vi "SLM 10-bit to 2xSLM 8-bit.vi"(1 "Array of voltages":i32[](array[numeric])) -> (0 "Array of SLM accepted voltages":u8[](array[numeric]))   [LabVIEW 2022 SP3]
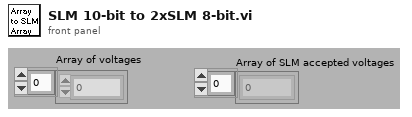
[diagram p1: front panel]
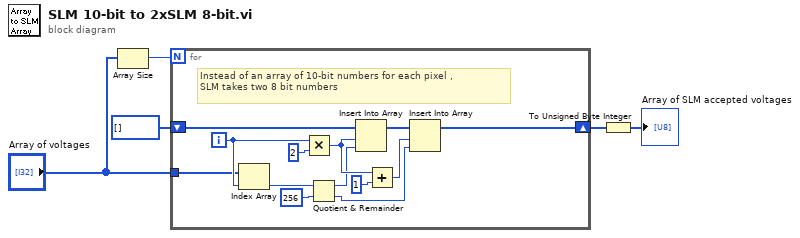
[diagram p0: block diagram]
diagram:
  n1 = Array Size(array="Array of voltages") -> (size(s)=w1:i32)
  n2 = for {
    N: w1 -> [_]
    shift-right: [w15] -> w4
    shift-left: i32[] [] -> [w18]
    tunnel: "Array of voltages" -> [w7]
    i -> [w9]
    # "Instead of an array of 10-bit numbers for each pixel ,\nSLM takes two 8 bit numbers"
    n3 = Index Array(array=w7, index=w9) -> (element=w6:i32)
    n4 = Multiply(x=w9, y=2) -> (x*y=w11:i32)
    n5 = Quotient & Remainder(x=w6, y=u16 256) -> (x-y*floor(x/y)=w8:i32, floor(x/y)=w10:i32)
    n6 = Insert Into Array(array=w18, index=w11, new element=w8) -> (w16:i32[])
    n7 = Add(x=w11, y=1) -> (x+y=w13:i32)
    n8 = Insert Into Array(array=w16, index=w13, new element=w10) -> (w15:i32[])
  }
  n9 = To Unsigned Byte Integer(number=w4) -> (unsigned 8bit integer=→"Array of SLM accepted voltages":u8[])
